vi "serial_monitor34.vi"(1 "ON\nOFF":bool caption="Init", 2 "Porta seriale":refnum<visa-resource-name>="COM12") -> ()   [LabVIEW 2014]
doc: "Lettura continua da porta seriale , INIT (true or false) della porta (9600, & bit, 1stop bit, EVEN)\nSalva su file\nFM&ADL aprile 2012"
uses:
  <vilib>/Instr/_visa.llb/VISA Configure Serial Port (Instr).vi
panel:
  in  "Baud rate":u32(ring)=115200 items=["9600"=9600, "14400"=14400, "19200"=19200, "38400"=38400, "57600"=57600, "115200"=115200]
  in  "SALVA I DATI SU FILE":bool=TRUE caption="ON\nOFF"
  out "N_dati":u32=389
  out "lung":i32=95232
  in  "stop":bool
  out "Number of Bytes at Serial Port":u32
  out "Dati trasmessi":string
  # "NO\nSI"
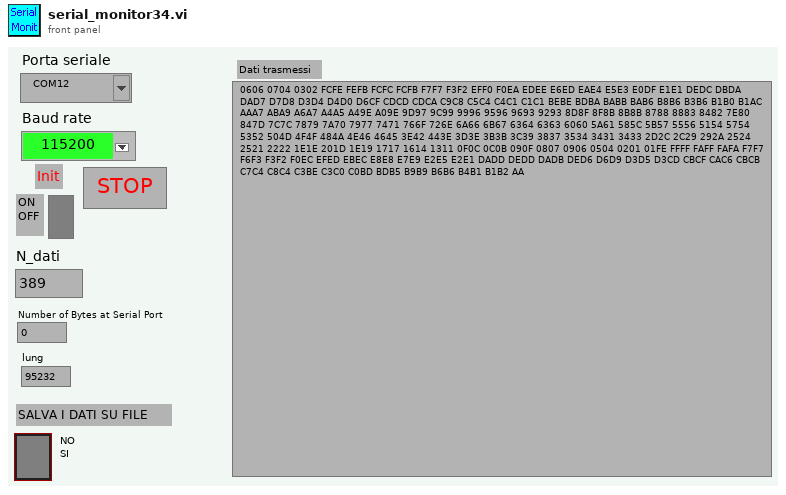
[diagram p1: front panel]
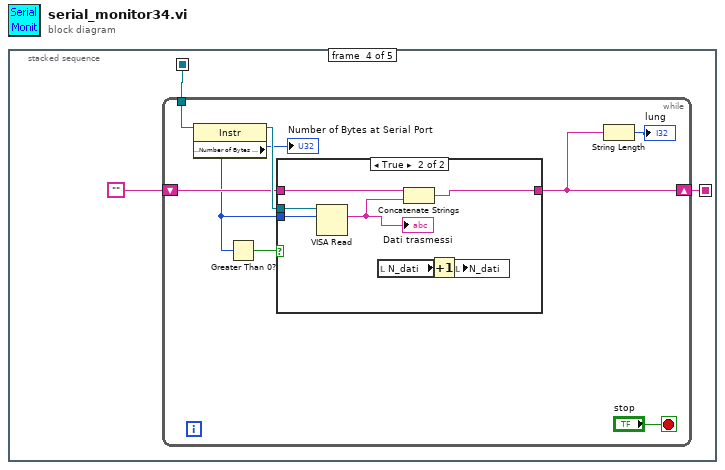
[diagram p0: block diagram]
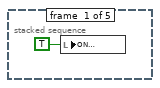
[diagram p2: hidden frame]
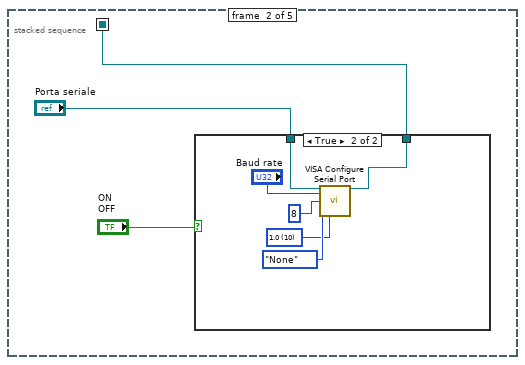
[diagram p3: hidden frame]
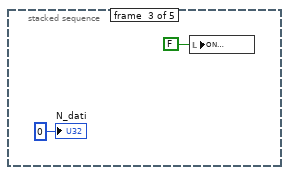
[diagram p5: hidden frame]
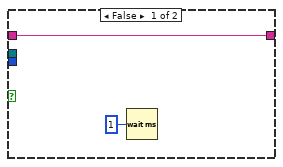
[diagram p6: hidden frame]
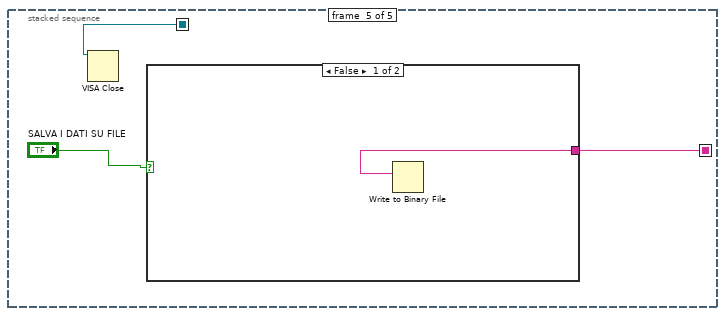
[diagram p7: hidden frame]
diagram:
  n1 = stacked-sequence {
    seq-local: [_ w2 _ _ _] -> [_ _ _ w16 w34]
    seq-local: [_ _ _ w14 _] -> [_ _ _ _ w35]
    frame #0 {
      n2 = local write "ON\nOFF"(TRUE ("ON\nOFF")) -> ()
    }
    frame #1 {
      n3 = case shown="True" "ON\nOFF" {
        tunnel: "Porta seriale" -> [w5 w7]
        tunnel: [w5 w6] -> w2
        frame False {
        }
        frame True {
          w8 = u16 10 items=["1.0"=10, "1.5"=15, "2.0"=20] ("stop bits (10: 1 bit)")
          n4 = call-poly "VISA Configure Serial Port"("VISA resource name"=w7, "baud rate (9600)"="Baud rate", "data bits (8)"=u16 8, "parity (0:none)"=enum16{"None", "Odd", "Even", "Mark", "Space"}."None", "stop bits (10: 1 bit)"=w8) -> ("VISA resource name out"=w6:refnum<visa-resource-name>)  [unwired: 2 in, 8 out]
        }
      }
    }
    frame #2 {
      n5 = local write "ON\nOFF"(FALSE ("ON\nOFF")) -> ()
      "N_dati" <- u32 0 ("N_dati")
    }
    frame #3 {
      n6 = while {
        tunnel: w16 -> [w23]
        shift-right: [w17] -> w14
        shift-left: "" -> [w21]
        stop <- "stop" stop-if-true
        n7 = property class="Instr"(reference=w23) -> (reference out=w22:refnum<visa-resource-name>, "Serial Settings:Number of Bytes at Serial Port"=w18:u32)  [unwired: 1 in, 1 out]
        "Number of Bytes at Serial Port" <- w18
        n8 = Greater Than 0?(x=w18) -> (x > 0?=w19:bool)
        n9 = case shown="True" w19 {
          tunnel: w22 -> [_ w33]
          tunnel: w18 -> [_ w32]
          tunnel: w21 -> [w26 w31]
          tunnel: [w26 w30] -> w17
          frame False {
            n10 = Wait (ms)(milliseconds to wait=u32 1) -> ()  [unwired: 1 out]
          }
          frame True {
            n11 = VISA Read(VISA resource name=w33, byte count=w32) -> (read buffer=w29:string)  [unwired: 1 in, 3 out]
            "Dati trasmessi" <- w29
            n12 = local read "N_dati"() -> (w28:u32)
            n13 = Concatenate Strings(w31, w29) -> (w30:string)
            n14 = Increment(x=w28) -> (x+1=w27:u32)
            n15 = local write "N_dati"(w27) -> ()
          }
        }
        n16 = String Length(string=w17) -> (length=→"lung":i32)
      }
    }
    frame #4 {
      n17 = VISA Close(VISA resource name=w34) -> ()  [unwired: 1 in, 1 out]
      n18 = case shown="False" "SALVA I DATI SU FILE" {
        tunnel: w35 -> [w37 _]
        frame False {
          n19 = Write to Binary File(data=w37) -> ()  [unwired: 2 in, 6 out]
        }
        frame True {
        }
      }
    }
  }
